vi "Round to Nearest (non-Banker).vi"(1 "Number":dbl) -> (0 "Rounded to Nearest":dbl)   [LabVIEW 2011]
panel:
  out "LabVIEW nearest integer value":dbl
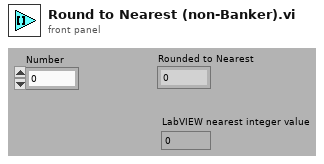
[diagram p1: front panel]
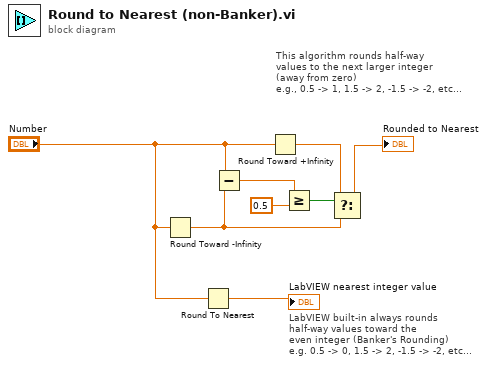
[diagram p0: block diagram]
diagram:
  # "This algorithm rounds half-way\nvalues to the next larger integer\n(away from zero)\ne.g., 0.5 -> 1, 1.5 -> 2, -1.5 -> -2, etc..."
  # "LabVIEW built-in always rounds\nhalf-way values toward the\neven integer (Banker's Rounding)\ne.g. 0.5 -> 0, 1.5 -> 2, -1.5 -> -2, etc..."
  n1 = Round Toward -Infinity(1:"Number") -> (0:w4:dbl)
  n2 = Round To Nearest(number="Number") -> (nearest integer value=→"LabVIEW nearest integer value":dbl)
  n3 = Subtract(x="Number", y=w4) -> (x-y=w8:dbl)
  n4 = Round Toward +Infinity(x="Number") -> (ceil(x): smallest int >= x=w5:dbl)
  n5 = Greater Or Equal?(x=w8, y=0.5) -> (x >= y?=w6:bool)
  n6 = Select(t=w5, s=w6, f=w4) -> (s? t:f=→"Rounded to Nearest":dbl)
